vi "Read RTM Dictionary.vi"(11 "Test Executive Builder View in":refnum<class "Test Executive Builder View.lvclass">) -> (2 "RTM Dictionary":variant, 3 "Test Executive Builder View out":refnum<class "Test Executive Builder View.lvclass">)   [LabVIEW 2017, in "Test Executive Builder View.lvclass"]
uses:
  <vilib>/gpm_packages/@cs/Test-executive-builder/Source/Test Executive Builder View/Test Executive Builder View/Test Executive Builder View.lvclass
  <vilib>/gpm_packages/@cs/Test-executive-builder/Source/Test Executive Builder View/Test Executive Builder View/Test Executive Builder View.lvclass/Test Executive Builder View.ctl
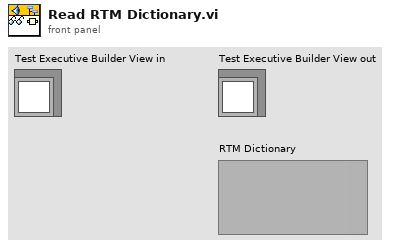
[diagram p1: front panel]
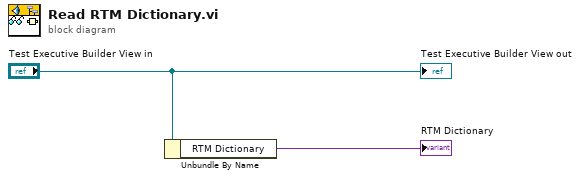
[diagram p0: block diagram]
diagram:
  n1 = Unbundle By Name("Test Executive Builder View in") -> ("RTM Dictionary"=→"RTM Dictionary":variant)
  "Test Executive Builder View out" <- "Test Executive Builder View in"
